vi "save_txt.vi"(0 "image":dbl[][](array[numeric]), 5 "image_info":T1={"file_path"=path "", "file_name"="", "image"=[], "image_size_xy"={"image_size_x_um"=1.0, "image_size_y_um"=1.0}, "pixel_dwell_time_ms"=1.0, "Laser_power_mW"=1.0, "pixel_size"=0.0, "tile_ij"={"tile_i"=0, "tile_j"=0}, "Objective"="", "ColorMarkers"=[], "timestamp"=timestamp(0 s since 1904-01-01), "micro-position-xyz"={"micro-position_x_mm"=1.0, "micro-position_y_mm"=1.0, "micro-position_z_mm"=1.0}, "zero_xyz"={"zero_x_mm"=0.0, "zero_y_mm"=0.0, "zero_z_mm"=0.0}, "nano-position-xyz"={"nano-position_x_V"=1.0, "nano-position_y_V"=1.0, "nano-position_z_V"=1.0}, "Kxyz"={"Kx_V/um"=1.0, "Ky_V/um"=1.0, "Kz_V/um"=1.0}}, 7 "run_number":i16 format="%03.0f") -> ()   [LabVIEW 2018]
uses:
  GLOBAL_VAR.vi
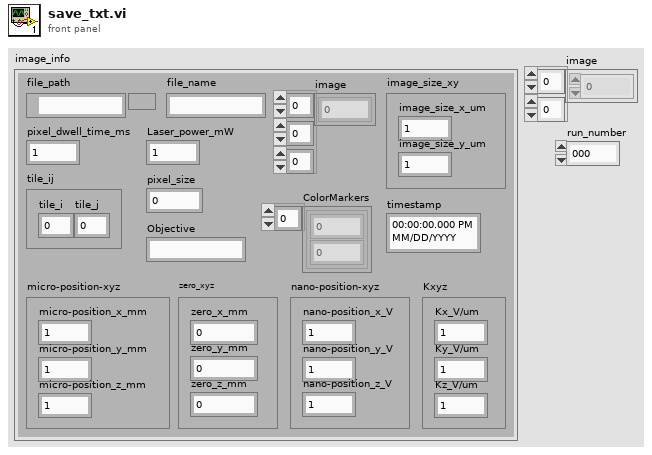
[diagram p1: front panel]
types:
  T1 = cluster{"file_path":path, "file_name":string, "image":dbl[][][], "image_size_xy":cluster{"image_size_x_um":sgl, "image_size_y_um":sgl}, "pixel_dwell_time_ms":sgl, "Laser_power_mW":sgl, "pixel_size":dbl, "tile_ij":cluster{"tile_i":i32, "tile_j":i32}, "Objective":string, "ColorMarkers":cluster{dbl, u32}[], "timestamp":timestamp, "micro-position-xyz":cluster{"micro-position_x_mm":sgl, "micro-position_y_mm":sgl, "micro-position_z_mm":sgl}, "zero_xyz":cluster{"zero_x_mm":dbl, "zero_y_mm":dbl, "zero_z_mm":dbl}, "nano-position-xyz":cluster{"nano-position_x_V":sgl, "nano-position_y_V":sgl, "nano-position_z_V":sgl}, "Kxyz":cluster{"Kx_V/um":sgl, "Ky_V/um":sgl, "Kz_V/um":sgl}}
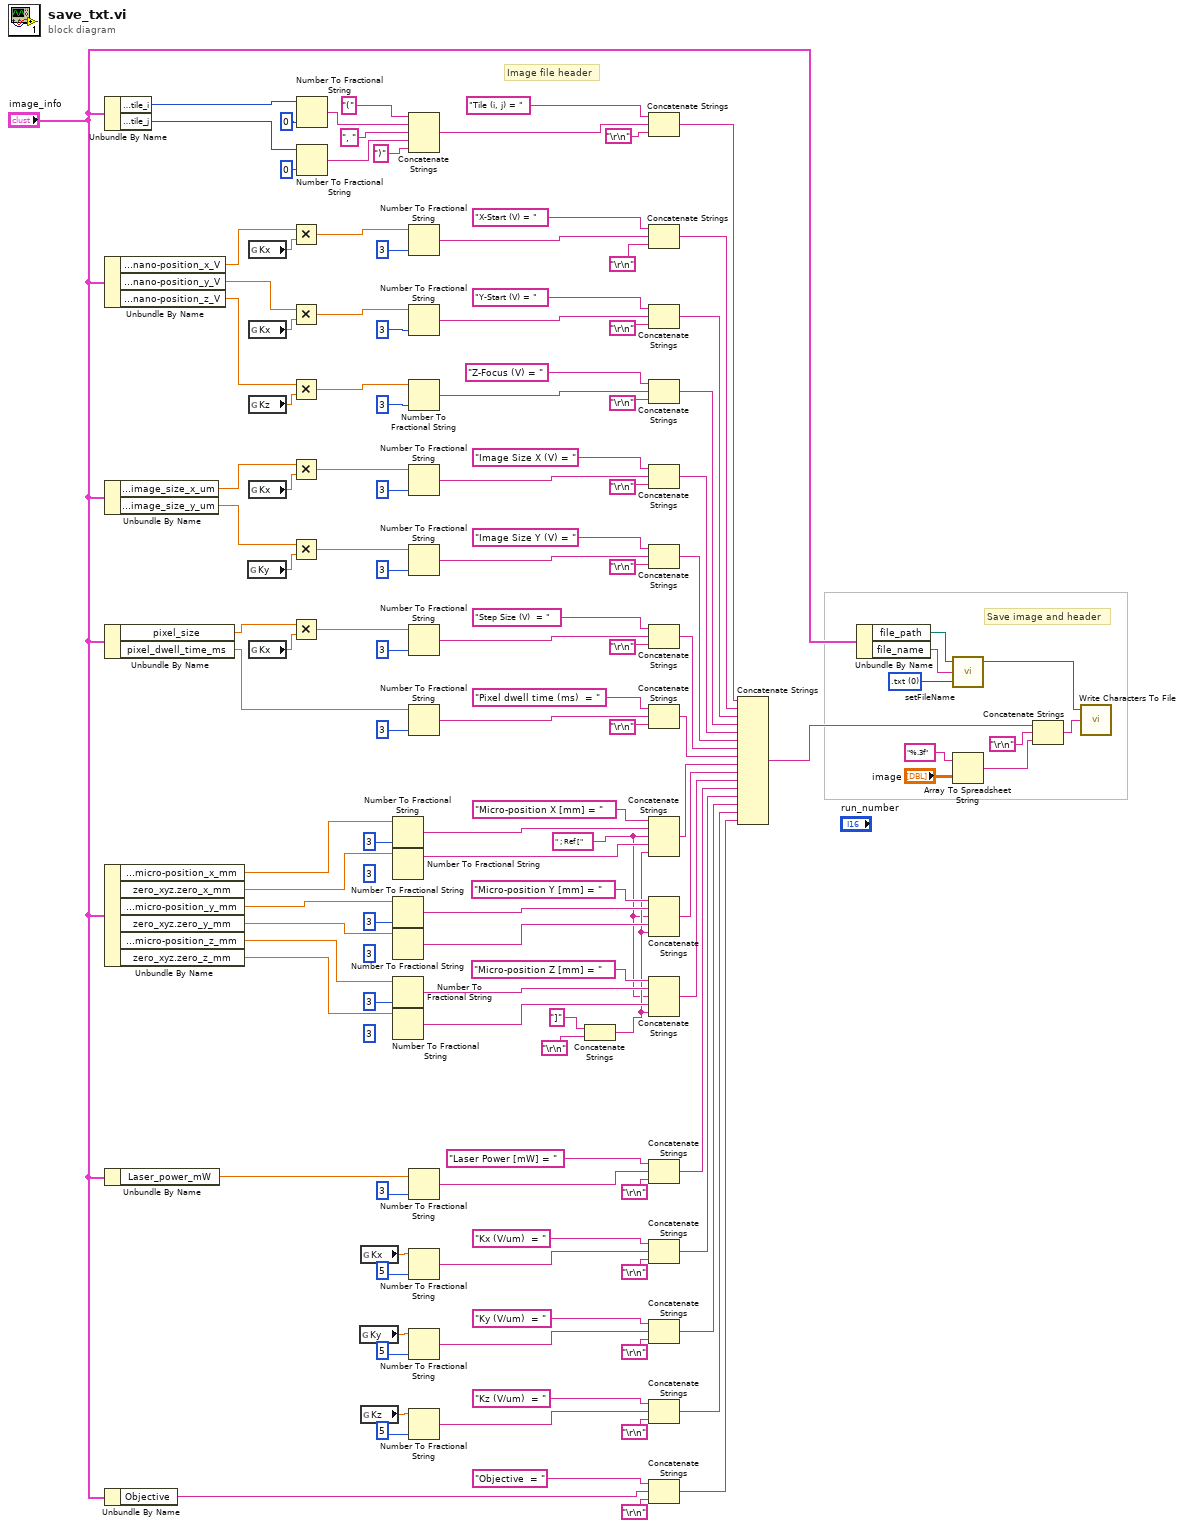
[diagram p0: block diagram]
diagram:
  w3 = u16 0 items=[".txt", ".tiff"] ("extension")
  (unwired) i16 3 ("precision (6)")
  (unwired) i16 3 ("precision (6)")
  (unwired) i16 3 ("precision (6)")
  w1 = " ; Ref [" ("string")
  # "Image file header"
  # "Save image and header"
  n1 = Unbundle By Name("image_info") -> ("tile_ij.tile_i"=w23:i32, "tile_ij.tile_j"=w22:i32)
  n2 = Unbundle By Name("image_info") -> ("nano-position-xyz.nano-position_x_V"=w21:sgl, "nano-position-xyz.nano-position_y_V"=w20:sgl, "nano-position-xyz.nano-position_z_V"=w19:sgl)
  n3 = Unbundle By Name("image_info") -> ("image_size_xy.image_size_x_um"=w18:sgl, "image_size_xy.image_size_y_um"=w17:sgl)
  n4 = Unbundle By Name("image_info") -> ("pixel_size"=w16:dbl, "pixel_dwell_time_ms"=w15:sgl)
  n5 = Unbundle By Name("image_info") -> ("micro-position-xyz.micro-position_x_mm"=w14:sgl, "zero_xyz.zero_x_mm"=w13:dbl, "micro-position-xyz.micro-position_y_mm"=w12:sgl, "zero_xyz.zero_y_mm"=w11:dbl, "micro-position-xyz.micro-position_z_mm"=w10:sgl, "zero_xyz.zero_z_mm"=w9:dbl)
  n6 = Unbundle By Name("image_info") -> ("Laser_power_mW"=w8:sgl)
  n7 = Unbundle By Name("image_info") -> ("Objective"=w7:string)
  n8 = global read "GLOBAL_VAR.vi" "Ky"() -> (w79:dbl)
  n9 = global read "GLOBAL_VAR.vi" "Kx"() -> (w88:dbl)
  n10 = global read "GLOBAL_VAR.vi" "Kx"() -> (w87:dbl)
  n11 = global read "GLOBAL_VAR.vi" "Kz"() -> (w29:dbl)
  n12 = global read "GLOBAL_VAR.vi" "Kx"() -> (w85:dbl)
  n13 = global read "GLOBAL_VAR.vi" "Kx"() -> (w75:dbl)
  n14 = Multiply(x=w21, y=w88) -> (x*y=w89:dbl)
  n15 = Multiply(x=w20, y=w87) -> (x*y=w86:dbl)
  n16 = Multiply(x=w19, y=w29) -> (x*y=w28:dbl)
  n17 = Multiply(x=w18, y=w85) -> (x*y=w84:dbl)
  n18 = Multiply(x=w17, y=w79) -> (x*y=w78:dbl)
  n19 = Multiply(x=w16, y=w75) -> (x*y=w74:dbl)
  n20 = Number To Fractional String(number=w23, precision (6)=i16 0) -> (F-format string=w122:string)  [unwired: 2 in]
  n21 = Number To Fractional String(number=w22, precision (6)=i16 0) -> (F-format string=w124:string)  [unwired: 2 in]
  n22 = global read "GLOBAL_VAR.vi" "Ky"() -> (w64:dbl)
  n23 = global read "GLOBAL_VAR.vi" "Kx"() -> (w69:dbl)
  n24 = global read "GLOBAL_VAR.vi" "Kz"() -> (w59:dbl)
  n25 = Number To Fractional String(number=w14, precision (6)=i16 3) -> (F-format string=w47:string)  [unwired: 2 in]
  n26 = Number To Fractional String(number=w13) -> (F-format string=w42:string)  [unwired: 3 in]
  n27 = Number To Fractional String(number=w12, precision (6)=i16 3) -> (F-format string=w50:string)  [unwired: 2 in]
  n28 = Number To Fractional String(number=w11) -> (F-format string=w41:string)  [unwired: 3 in]
  n29 = Number To Fractional String(number=w10, precision (6)=i16 3) -> (F-format string=w44:string)  [unwired: 2 in]
  n30 = Number To Fractional String(number=w9) -> (F-format string=w40:string)  [unwired: 3 in]
  n31 = Concatenate Strings("(", w122, ", ", w124, ")") -> (w90:string)
  n32 = Number To Fractional String(number=w89, precision (6)=i16 3) -> (F-format string=w118:string)  [unwired: 2 in]
  n33 = Number To Fractional String(number=w86, precision (6)=i16 3) -> (F-format string=w114:string)  [unwired: 2 in]
  n34 = Number To Fractional String(number=w28, precision (6)=i16 3) -> (F-format string=w32:string)  [unwired: 2 in]
  n35 = Number To Fractional String(number=w84, precision (6)=i16 3) -> (F-format string=w110:string)  [unwired: 2 in]
  n36 = Number To Fractional String(number=w78, precision (6)=i16 3) -> (F-format string=w82:string)  [unwired: 2 in]
  n37 = Number To Fractional String(number=w74, precision (6)=i16 3) -> (F-format string=w106:string)  [unwired: 2 in]
  n38 = Number To Fractional String(number=w15, precision (6)=i16 3) -> (F-format string=w100:string)  [unwired: 2 in]
  n39 = Number To Fractional String(number=w8, precision (6)=i16 3) -> (F-format string=w95:string)  [unwired: 2 in]
  n40 = Number To Fractional String(number=w69, precision (6)=i16 5) -> (F-format string=w72:string)  [unwired: 2 in]
  n41 = Number To Fractional String(number=w64, precision (6)=i16 5) -> (F-format string=w67:string)  [unwired: 2 in]
  n42 = Number To Fractional String(number=w59, precision (6)=i16 5) -> (F-format string=w62:string)  [unwired: 2 in]
  n43 = Concatenate Strings("]" ("string"), "\r\n") -> (w37:string)
  n44 = Concatenate Strings("Tile (i, j) = " ("string"), w90, "\r\n") -> (w27:string)
  n45 = Concatenate Strings("X-Start (V) = " ("string"), w118, "\r\n") -> (w26:string)
  n46 = Concatenate Strings("Y-Start (V) = " ("string"), w114, "\r\n") -> (w25:string)
  n47 = Concatenate Strings("Z-Focus (V) = " ("string"), w32, "\r\n") -> (w24:string)
  n48 = Concatenate Strings("Image Size X (V) = " ("string"), w110, "\r\n") -> (w103:string)
  n49 = Concatenate Strings("Image Size Y (V) = " ("string"), w82, "\r\n") -> (w76:string)
  n50 = Concatenate Strings("Step Size (V)  = " ("string"), w106, "\r\n") -> (w77:string)
  n51 = Concatenate Strings("Pixel dwell time (ms)  = " ("string"), w100, "\r\n") -> (w98:string)
  n52 = Concatenate Strings("Micro-position X [mm] = ", w47, w1, w42, w37) -> (w36:string)
  n53 = Concatenate Strings("Micro-position Y [mm] = ", w50, w1, w41, w37) -> (w35:string)
  n54 = Concatenate Strings("Micro-position Z [mm] = ", w44, w1, w40, w37) -> (w34:string)
  n55 = Concatenate Strings("Laser Power [mW] = " ("string"), w95, "\r\n") -> (w93:string)
  n56 = Concatenate Strings("Kx (V/um)  = " ("string"), w72, "\r\n") -> (w56:string)
  n57 = Concatenate Strings("Ky (V/um)  = " ("string"), w67, "\r\n") -> (w55:string)
  n58 = Concatenate Strings("Kz (V/um)  = " ("string"), w62, "\r\n") -> (w54:string)
  n59 = Concatenate Strings("Objective  = " ("string"), w7, "\r\n") -> (w53:string)
  n60 = Concatenate Strings(w27, w26, w25, w24, w103, w76, w77, w98, w36, w35, w34, w93, w56, w55, w54, w53) -> (w91:string)
  n61 = Unbundle By Name("image_info") -> ("file_path"=w5:path, "file_name"=w4:string)
  n62 = call "setFileName.vi"("extension"=w3, "file_name"=w4, "base_path"=w5) -> ("path_filename"=w2:path)  [unwired: 2 in]
  n63 = Array To Spreadsheet String(array="image", 3:"%.3f" ("format string")) -> (spreadsheet string=w130:string)  [unwired: 1 in]
  n64 = Concatenate Strings(w91, "\r\n", w130) -> (w128:string)
  n65 = call <vilib>:"Write Characters To File.vi"("character string"=w128, "file path (dialog if empty)"=w2) -> ()  [unwired: 3 in, 1 out]
